vi "FlukeTime2TS.vi"(1 "Fluke Time":string) -> (0 "timestamp out":timestamp format="%^<%.3X\n%x>T")   [LabVIEW 2014]
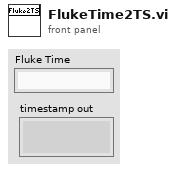
[diagram p1: front panel]
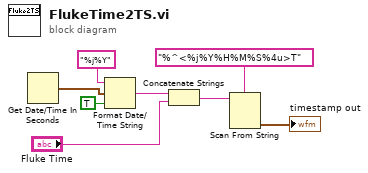
[diagram p0: block diagram]
diagram:
  n1 = Get Date/Time In Seconds() -> (seconds since 1Jan1904=w7:timestamp)
  n2 = Format Date/Time String(time format string (%c)="%j%Y", seconds (now)=w7, UTC format=TRUE) -> (date/time string=w5:string)
  n3 = Concatenate Strings(w5, "Fluke Time") -> (w3:string)
  n4 = Scan From String(format string="%^<%j%Y%H%M%S%4u>T", input string=w3) -> (output 1=→"timestamp out":timestamp)  [unwired: 3 in, 3 out]
